vi "Pfeiffer-RVC300.set gas flow.vi"(0 "i ref in":refnum<vi>, 3 "gas_flow":dbl format="%.2f", 5 "error in (no error)":errorcluster) -> (14 "i ref out":refnum<vi>, 18 "gas_flow_out":dbl format="%.2f", 19 "error out":errorcluster)   [LabVIEW 2014, in "Pfeiffer-RVC300.lvlib"]
doc: "This is the constructor of a class.\n\nLicense Agreement for this software:\n\nCopyright (C)\nGesellschaft für Schwerionenforschung, GSI\nPlanckstr. 1\n64291 Darmstadt\nGermany\n\nContact: D.Beck@gsi.de \n\nThis program is free software; you can redistribute it and/or modify it under the terms of the \nGNU General Public License as published by the Free Software Foundation; either version 2 of \nthe license, or (at your option) any later version.\n\nThis program is distributed in the hope that it will be useful, but WITHOUT ANY WARRANTY; \nwithout even the implied warranty of MERCHANTABILITY or FITNESS FOR A PARTICULAR PURPOSE. See the GNU General License for more details (http://www.gnu.org).\n\nGesellschaft für Schwerionenforschung, GSI\nPlanckstr. 1, 64291 Darmstadt, Germany\nFor all questions and ideas contact: M.Richter@gsi.de, H.Brand@gsi.de or D.Beck@gsi.de.\nLast update: 16-JUN-2004"
uses:
  Pfeiffer-RVC300.lvlib
  CS_Core/CSSystem/CoreDefs/CoreDefs.error_type.ctl
  CS_Core/CSSystem/CoreLib/CoreLib.lvlib
  instr.lib/RVC300/RVC-300.lvlib
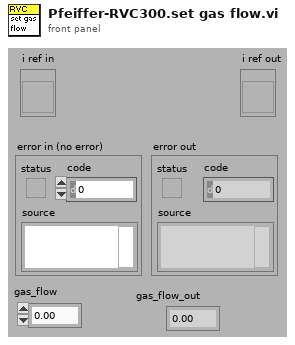
[diagram p1: front panel]
types:
  T1 = typedef "CoreDefs.error_type.ctl" = enum16{"no error", "can't load process", "can't unload process", "process does not exist", "can't install process", "can't remove process", "unknown function", "time out", "can't execute function", "duplicate queue name", "super not found", "caller queue invalid", "can't ping process", "unknown error", "VISA Error", "VISA timeout", "GPIB timeout", "GPIB error", "communication error", "data type mismatch", "can't read data from OPC server", "can't write data to OPC server", "OET error", "function not implemented", "process already exists", "invalid Shared Variable name", "error writing Shared Variable", "error reading Shared Variable", "invalid client name", "corrupt database", "unknown class", "call not authorized", "parameter out of range", "OET timeout: can't get data to modify", "invalid queue name", "requested operation incompatible with current state", "event undefined", "event disabled", "state undefined", "caller is not a friend", "EventBuilder: bad eventID", "EventBuilder: no DAQ devices", "a thread must not stop itself", "UNUSED ELEMENT4", "DiscArchiver: eventData incomplete", "DiscArchiver: eventData does not belong to run", "DiscArchiver: can't open file", "DiscArchiver: can't write to file", "DiscArchiver: available disc space low", "can't acquire semaphore", "error reading data from database", "notifier object is not existing", "can't register process", "can't unregister process", "illegal event type", "object disabled", "object already exists", "can't change state", "Instrument not found", "no connection to remote node", "invalid reference", "N/A", "UNUSED ELEMENT 1", "element not found", "illegal TCP/IP connection detected", "object does not exist", "invalid access ID", "unknown CS system", "invalid privilige", "unsupported data type", "unsupported server type", "IO server already exists", "Shared Variable already exists"}
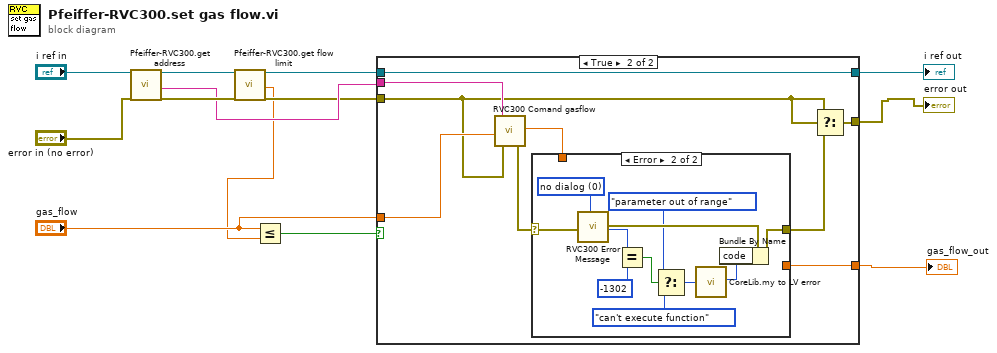
[diagram p0: block diagram]
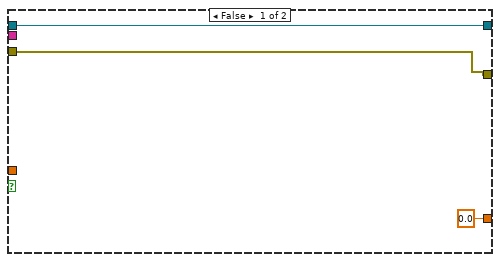
[diagram p2: hidden frame]
diagram:
  n1 = call "Pfeiffer-RVC300.get address.vi"("i ref in"="i ref in", "error in (no error)"="error in (no error)") -> ("i ref out"=w9:refnum<vi>, "address"=w7:string, "error out"=w8:errorcluster)  [unwired: 15 in]
  n2 = call "Pfeiffer-RVC300.get flow limit.vi"("i ref in"=w9, "error in (no error)"=w8) -> ("i ref out"=w4:refnum<vi>, "flow_limit"=w1:dbl, "error out"=w3:errorcluster)  [unwired: 15 in]
  n3 = Less Or Equal?(x="gas_flow", y=w1) -> (x <= y?=w2:bool)
  n4 = case shown="True" w2 {
    tunnel: w7 -> [_ w25]
    tunnel: "gas_flow" -> [_ w24]
    tunnel: w3 -> [w15 w22]
    tunnel: [w15 w20] -> w11
    tunnel: [0.0 ("Gas Flow readout [mbarl/s]") w18] -> w5
    tunnel: w4 -> [w16 w17]
    tunnel: [w16 w17] -> w10
    frame False {
    }
    frame True {
      n5 = call "RVC300 Comand gasflow.vi"("Flow value [ x.xxEsxx}mbarl/s"=w24, "RVC300 VISA Resource Name"=w25, "error in (no error)"=w22) -> ("error out"=w23:errorcluster, "Gas Flow readout [mbarl/s]"=w19:dbl)  [unwired: 13 in, 2 out]
      n6 = case shown="Error" w23 {
        selector: w23 -> [w26 w37]
        tunnel: [w26 w34] -> w21
        tunnel: w19 -> [w27 _]
        tunnel: [w27 _] -> w18
        frame No Error {
        }
        frame Error {
          w38 = u16 0 items=["no dialog", "OK message", "continue or stop message"] ("type of dialog (OK msg:1)")
          n7 = call "RVC300 Error Message.vi"("error in (no error)"=w37, "type of dialog (OK msg:1)"=w38) -> ("error out"=w36:errorcluster, "code out"=w32:i32)  [unwired: 12 in, 4 out]
          n8 = Equal?(x=w32, y=-1302) -> (x = y?=w33:bool)
          n9 = Select(t=CoreDefs.error_type."parameter out of range" ("ErrorTypes"), s=w33, f=CoreDefs.error_type."can't execute function" ("ErrorTypes")) -> (s? t:f=w28:T1)
          n10 = call "CoreLib.my to LV error.vi"("ErrorTypes"=w28) -> ("LV error code"=w35:i32)  [unwired: 17 in, 1 out]
          n11 = Bundle By Name(cluster=w36, "code"=w35) -> (w34:errorcluster)
        }
      }
      n12 = Select(t=w22, s=w22, f=w21) -> (s? t:f=w20:errorcluster)
    }
  }
  "error out" <- w11
  "i ref out" <- w10
  "gas_flow_out" <- w5
